vi "Get Instrument VI Paths.vi"(8 "error in":errorcluster) -> (0 "error out":errorcluster, 3 "instr vi paths[]":path[](array[path]))   [LabVIEW 2021, in "Converter Reusables.lvlib"]
uses:
  Converter Reusables.lvlib
  TypeDefs/Dictionary States.ctl
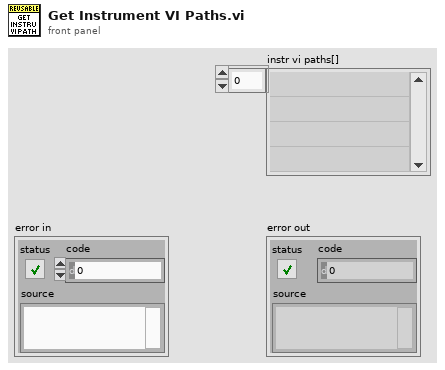
[diagram p1: front panel]
types:
  T1 = typedef "Converter Reusables.lvlib/Dictionary States.ctl" = enum16{"Set", "Get", "Delete", "Delete All"}
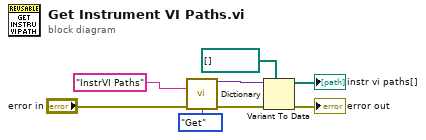
[diagram p0: block diagram]
diagram:
  n1 = call "Dictionary.vi"("key"="InstrVI Paths" ("Key"), "error in"="error in", "dict states"=Dictionary_States."Get" ("Dict States")) -> ("variant out"=w4:variant, "error out"=w5:errorcluster)  [unwired: 11 in]
  n2 = Variant To Data(error in=w5, type=path[] [], Variant=w4) -> (data=→"instr vi paths[]":path[], error out=→"error out":errorcluster)
